vi "Variant To String.vi"(2 "error in (no error)":errorcluster, 3 "Variant":variant) -> (0 "error out":errorcluster, 1 "String":string)   [LabVIEW 2023, in "Logging.lvlib"]
uses:
  Logging.lvlib
  <vilib>/Utility/Data Type/NI_Data Type.lvlib
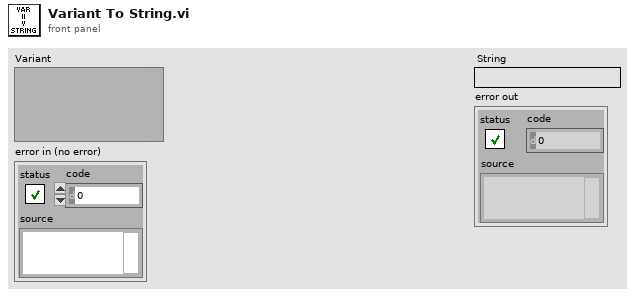
[diagram p1: front panel]
types:
  T1 = typedef "NI_Data Type.lvlib/Data Type.ctl" = enum8{"Invalid Type", "Void", "I8", "I16", "I32", "I64", "U8", "U16", "U32", "U64", "Single Float", "Double Float", "Extended Float", "Single Complex", "Double Complex", "Extended Complex", "Enum U8", "Enum U16", "Enum U32", "Enum U64", "Single Float With Unit", "Double Float With Unit", "Extended Float With Unit", "Single Complex with Unit", "Double Complex with Unit", "Extended Complex with Unit", "Boolean", "String", "Path", "Picture", "Tag", "Array", "Cluster", "Variant", "LV Variant", "Waveform", "Timestamp", "Digital Waveform", "Digital Data", "ExpressData", "Refnum", "External Data", "VI", "Poly VI", "LabVIEW Class Instance", "Fixed Point", "Set Collection", "Map Collection"}
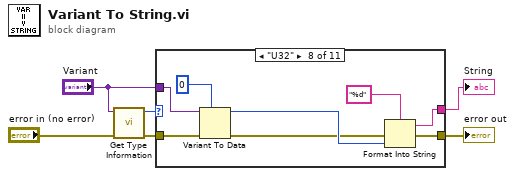
[diagram p0: block diagram]
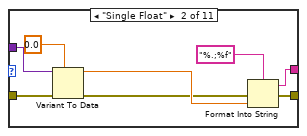
[diagram p3: hidden frame]
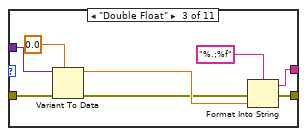
[diagram p4: hidden frame]
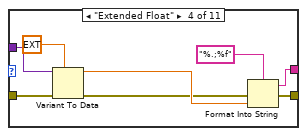
[diagram p5: hidden frame]
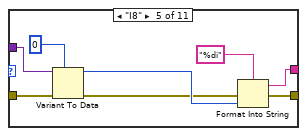
[diagram p6: hidden frame]
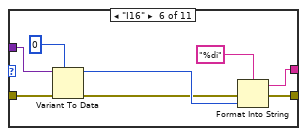
[diagram p7: hidden frame]
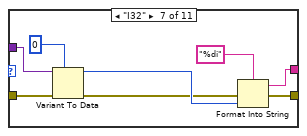
[diagram p8: hidden frame]
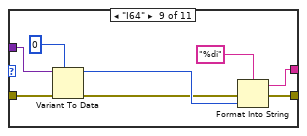
[diagram p9: hidden frame]
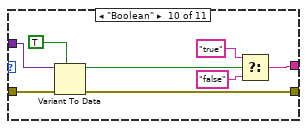
[diagram p10: hidden frame]
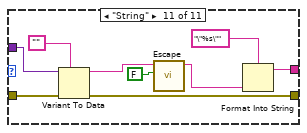
[diagram p11: hidden frame]
diagram:
  n1 = call <vilib>:"Get Type Information.vi"("error in (no error)"="error in (no error)", "variant"="Variant") -> ("error out"=w5:errorcluster, "type"=w6:T1)  [unwired: 5 in, 3 out]
  n2 = case shown="\"U32\"" w6 {
    tunnel: "Variant" -> [_ w15 w23 w31 w39 w47 w55 w63 w71 w79 w88]
    tunnel: w5 -> [w7 w11 w19 w27 w35 w43 w51 w60 w67 w77 w86]
    tunnel: [_ w9 w17 w25 w33 w41 w49 w58 w65 w74 w82] -> w4
    tunnel: [w7 w8 w16 w24 w32 w40 w48 w57 w64 w72 w80] -> w1
    frame Default {
    }
    frame "Single Float" {
      n3 = Variant To Data(error in=w11, type=sgl 0.0, Variant=w15) -> (data=w13:sgl, error out=w12:errorcluster)
      n4 = Format Into String(format string="%.;%f", error in=w12, w13) -> (resulting string=w9:string, error out=w8:errorcluster)  [unwired: 1 in]
    }
    frame "Double Float" {
      n5 = Variant To Data(error in=w19, type=0.0, Variant=w23) -> (data=w21:dbl, error out=w20:errorcluster)
      n6 = Format Into String(format string="%.;%f", error in=w20, w21) -> (resulting string=w17:string, error out=w16:errorcluster)  [unwired: 1 in]
    }
    frame "Extended Float" {
      n7 = Variant To Data(error in=w27, type=ext 0.0, Variant=w31) -> (data=w29:ext, error out=w28:errorcluster)
      n8 = Format Into String(format string="%.;%f", error in=w28, w29) -> (resulting string=w25:string, error out=w24:errorcluster)  [unwired: 1 in]
    }
    frame "I8" {
      n9 = Variant To Data(error in=w35, type=i8 0, Variant=w39) -> (data=w37:i8, error out=w36:errorcluster)
      n10 = Format Into String(format string="%di", error in=w36, w37) -> (resulting string=w33:string, error out=w32:errorcluster)  [unwired: 1 in]
    }
    frame "I16" {
      n11 = Variant To Data(error in=w43, type=i16 0, Variant=w47) -> (data=w45:i16, error out=w44:errorcluster)
      n12 = Format Into String(format string="%di", error in=w44, w45) -> (resulting string=w41:string, error out=w40:errorcluster)  [unwired: 1 in]
    }
    frame "I32" {
      n13 = Variant To Data(error in=w51, type=0, Variant=w55) -> (data=w53:i32, error out=w52:errorcluster)
      n14 = Format Into String(format string="%di", error in=w52, w53) -> (resulting string=w49:string, error out=w48:errorcluster)  [unwired: 1 in]
    }
    frame "U32" {
      n15 = Variant To Data(error in=w60, type=u32 0 ("notification"), Variant=w63) -> (data=w62:u32, error out=w61:errorcluster)
      n16 = Format Into String(format string="%d", error in=w61, w62) -> (resulting string=w58:string, error out=w57:errorcluster)  [unwired: 1 in]
    }
    frame "I64" {
      n17 = Variant To Data(error in=w67, type=i64 0, Variant=w71) -> (data=w69:i64, error out=w68:errorcluster)
      n18 = Format Into String(format string="%di", error in=w68, w69) -> (resulting string=w65:string, error out=w64:errorcluster)  [unwired: 1 in]
    }
    frame "Boolean" {
      n19 = Variant To Data(error in=w77, type=TRUE, Variant=w79) -> (data=w76:bool, error out=w72:errorcluster)
      n20 = Select(t="true", s=w76, f="false") -> (s? t:f=w74:string)
    }
    frame "String" {
      n21 = Variant To Data(error in=w86, type="", Variant=w88) -> (data=w85:string, error out=w80:errorcluster)
      n22 = call "Escape.vi"("Escape Equal Sign"=FALSE, "String in"=w85) -> ("String out"=w83:string)  [unwired: 9 in]
      n23 = Format Into String(format string="\"%s\"", w83) -> (resulting string=w82:string)  [unwired: 2 in, 1 out]
    }
  }
  "String" <- w4
  "error out" <- w1
